vi "grSim_ReplacementTester.vi"(0 "Generate new random points":bool, 1 "IA State":T3, 2 "Atacando contra?":bool, 3 "Test Attacker":bool, 4 "id":i32, 5 "Field defense":i32[](array[numeric]), 6 "Test Mode On":bool, 7 "Number of Points":i32, 10 "Modulo Velocidade":dbl format="%#_13g", 11 "Test Passe":bool, 12 "reset":bool, 13 "Replace Robots":bool) -> (14 "grSim replacement":cluster{"robots":T1[], "ball":T2}, 15 "Replace active":bool, 18 "kick num":i32, 19 "Completed Generation":bool)   [LabVIEW 2017]
uses:
  Core/AI Input.ctl
  Core/AI Robot.ctl
  Intel/Functions Enum.ctl
  Intel/AttackerStates.ctl
  Path Planning/RRT/PathDests.ctl
  Path Planning/RRT/PathDest.ctl
  Core/AI Ball.ctl
  Core/Field Size.ctl
  Core/AI Judge.ctl
  Intel/Command Enum.ctl
  Util/Events/Events.ctl
  grSim RobotReplacement.ctl
  grSim_BallReplacement.ctl
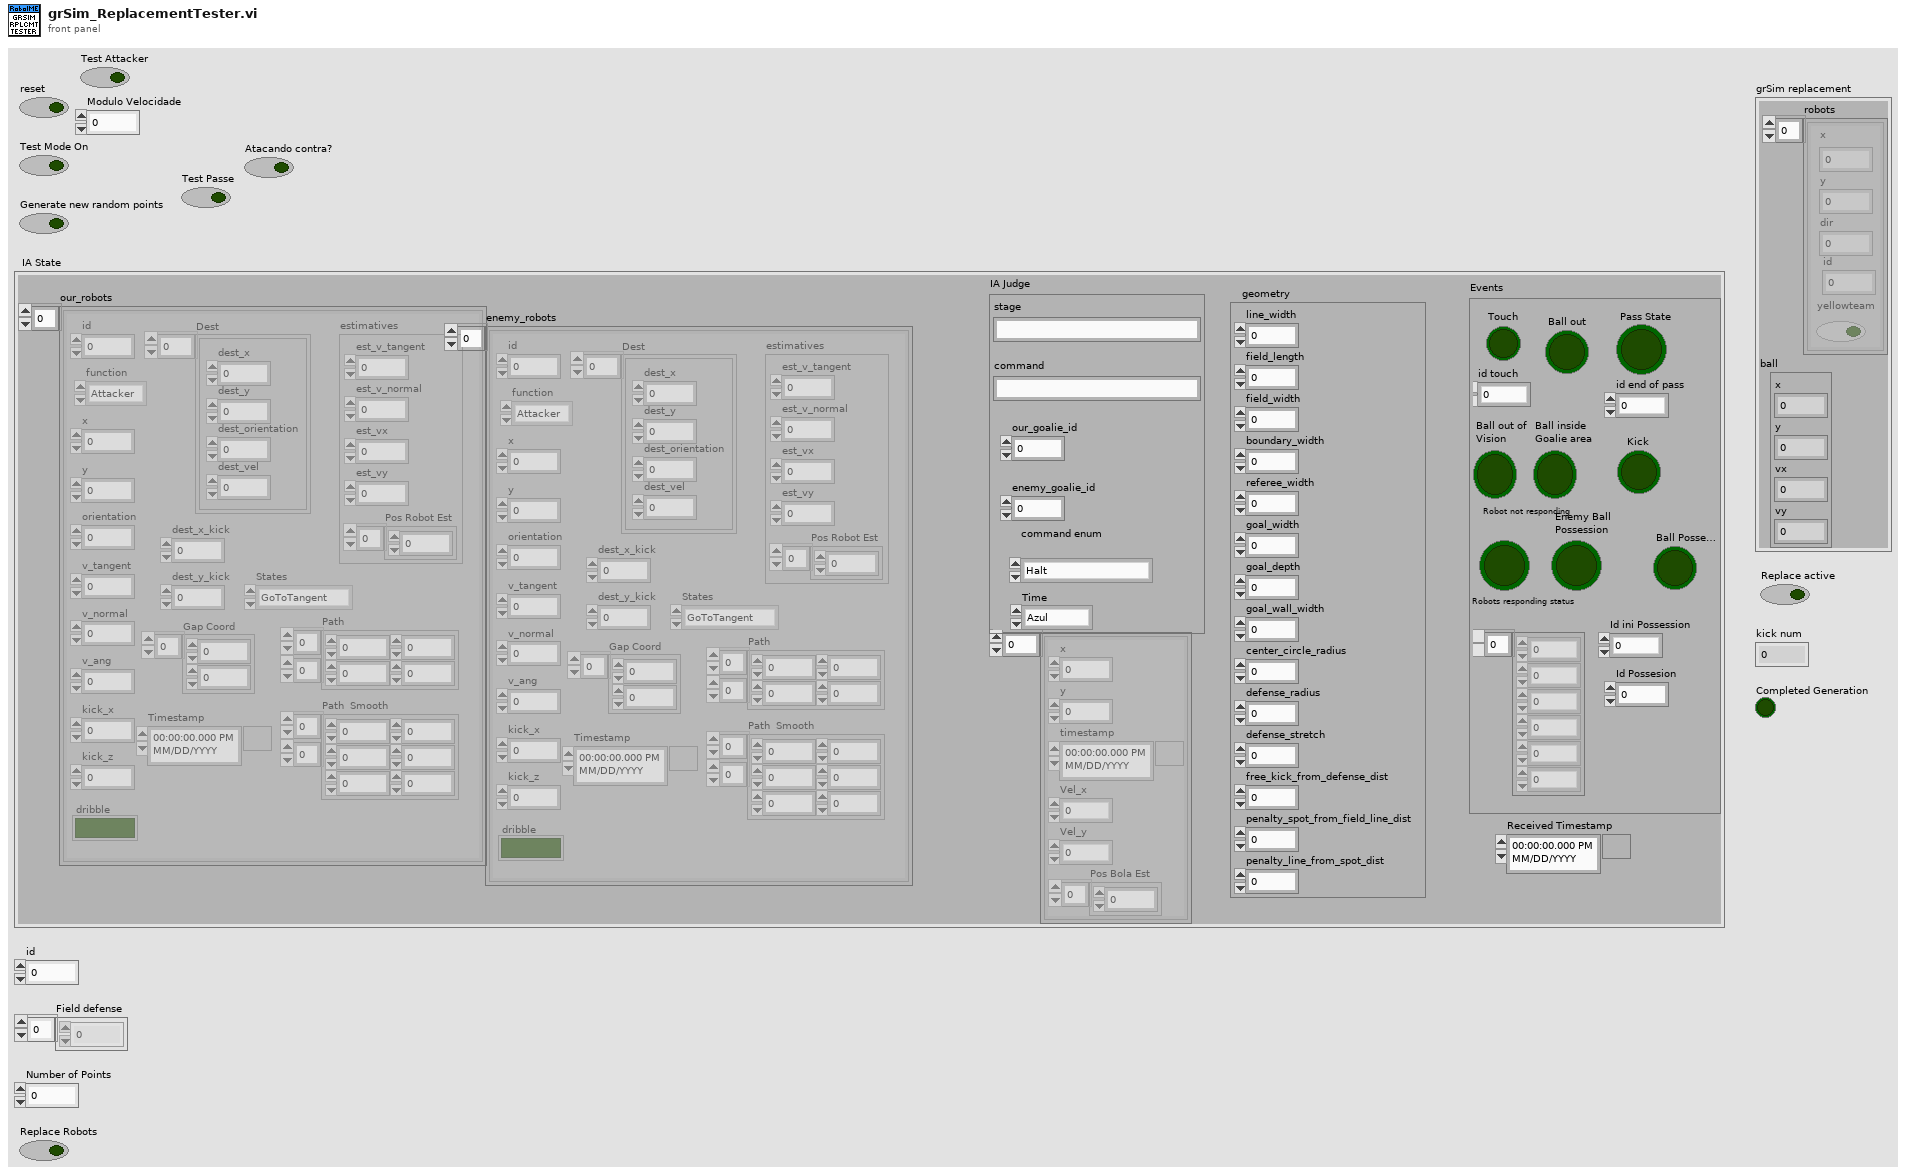
[diagram p1: front panel]
types:
  T1 = typedef "grSim RobotReplacement.ctl" = cluster{"x":dbl, "y":dbl, "dir":dbl, "yellowteam":bool, "id":u32}
  T2 = typedef "grSim_BallReplacement.ctl" = cluster{"x":dbl, "y":dbl, "vx":dbl, "vy":dbl}
  T3 = typedef "AI Input.ctl" = cluster{"our_robots":T4[], "enemy_robots":T4[], "balls":T9[], "geometry":T10, "IA Judge":T11, "Received Timestamp":timestamp, "Events":T13}
  T4 = typedef "AI Robot.ctl" = cluster{"id":u32, "function":T5, "x":dbl, "y":dbl, "orientation":dbl, "v_tangent":dbl, "v_normal":dbl, "v_ang":dbl, "kick_x":dbl, "kick_z":dbl, "dribble":bool, "Timestamp":timestamp, "estimatives":cluster{"est_v_tangent":dbl, "est_v_normal":dbl, "est_vx":dbl, "est_vy":dbl, "Pos Robot Est":dbl[]}, "dest_x_kick":dbl, "dest_y_kick":dbl, "Gap Coord":dbl[], "States":T6, "Path ":dbl[][], "Path  Smooth":dbl[][], "Dest":T7}
  T5 = typedef "Functions Enum.ctl" = enum16{"Attacker", "Goalie", "Defender", "Striker", "Goto 0", "Dummy", "Kicker", "ZigZag"}
  T6 = typedef "AttackerStates.ctl" = enum16{"Pass", "GoToTangent", "BallGetting", "GoToKick", ""}
  T7 = typedef "PathDests.ctl" = T8[]
  T8 = typedef "PathDest.ctl" = cluster{"dest_x":dbl, "dest_y":dbl, "dest_orientation":dbl, "dest_vel":dbl}
  T9 = typedef "AI Ball.ctl" = cluster{"x":dbl, "y":dbl, "timestamp":timestamp, "Vel_x":dbl, "Vel_y":dbl, "Pos Bola Est":dbl[]}
  T10 = typedef "Field Size.ctl" = cluster{"line_width":u32, "field_length":u32, "field_width":u32, "boundary_width":u32, "referee_width":u32, "goal_width":u32, "goal_depth":u32, "goal_wall_width":u32, "center_circle_radius":u32, "defense_radius":u32, "defense_stretch":u32, "free_kick_from_defense_dist":u32, "penalty_spot_from_field_line_dist":u32, "penalty_line_from_spot_dist":u32}
  T11 = typedef "AI Judge.ctl" = cluster{"stage":string, "command":string, "our_goalie_id":dbl, "enemy_goalie_id":dbl, "command enum":T12, "Time":enum16{"Azul", "Amarelo"}}
  T12 = typedef "Command Enum.ctl" = enum16{"Halt", "Stop", "Force Start", "PKA Normal Start", "Prepare Kickoff Ally", "PKE Normal Start", "Prepare Kickoff Enemy", "Prepare Penalty Ally", "PPA Normal Start", "Prepare Penalty Enemy", "PPE Normal Start", "Direct Free Enemy", "Direct Free Ally", "Indirect Free Enemy", "Indirect Free Ally", "Timeout Enemy", "Timeout Ally", "Goal Enemy", "Goal Ally", "Ball Placement Enemy", "Ball Placement Ally", "Normal Half Time", "Extra Time Break", "Extra Half Time", "None", "Post Game"}
  T13 = typedef "Events.ctl" = cluster{"Touch":bool, "Ball out":bool, "id touch":dbl, "Ball out of \nVision":bool, "Ball inside \nGoalie area":bool, "Robot not responding":bool, "Robots responding status":dbl[], "Enemy Ball \nPossession":bool, "Pass State":bool, "id end of pass":dbl, "Kick":bool, "Id ini Possession":dbl, "Ball Possesion":bool, "Id Possesion":dbl}
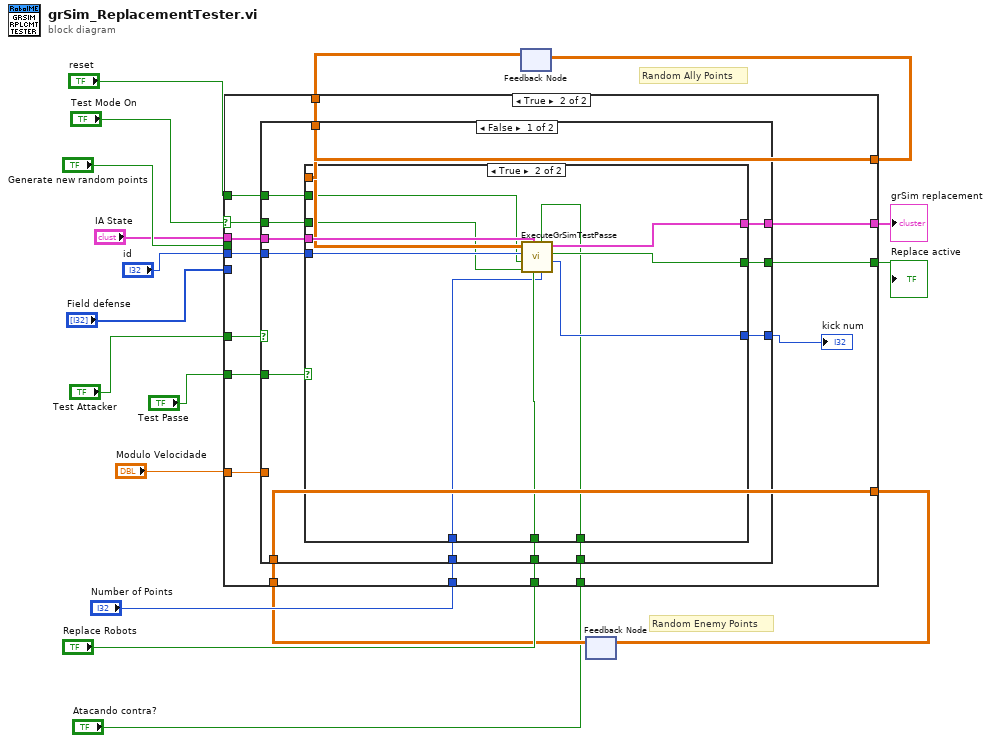
[diagram p0: block diagram]
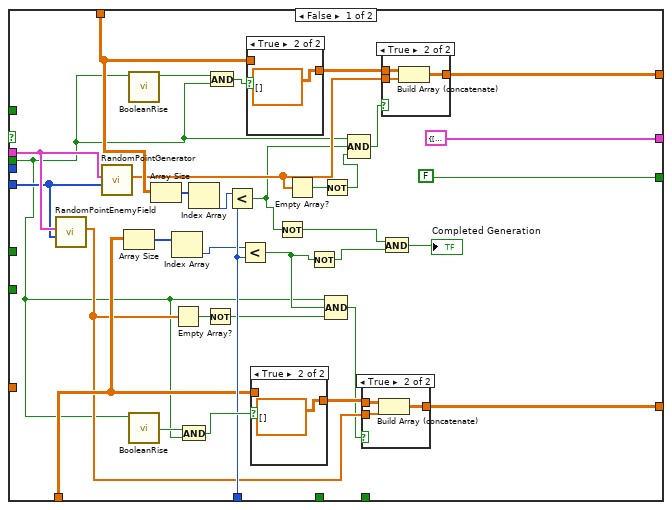
[diagram p2: hidden frame]
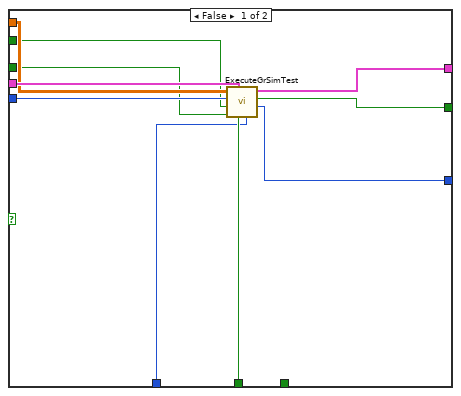
[diagram p7: hidden frame]
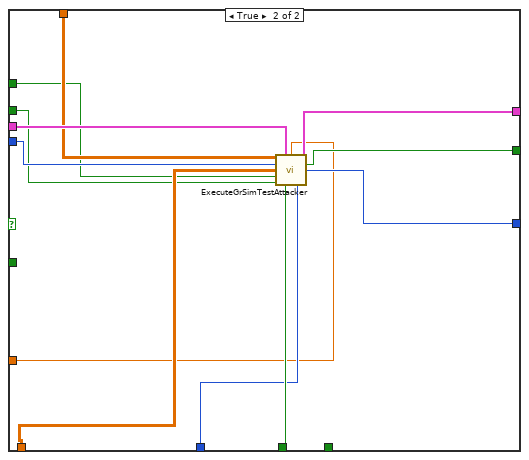
[diagram p8: hidden frame]
diagram:
  # "Random Enemy Points"
  # "Random Ally Points"
  n1 = feedback #1() -> (w14:dbl[][])  [unwired: 1 in]
  n2 = feedback #2() -> (w5:dbl[][])  [unwired: 1 in]
  n3 = case shown="True" "Test Mode On" {
    selector: "Test Mode On" -> [_ w73]
    tunnel: [cluster{"robots":T1[], "ball":T2} {"robots"=[], "ball"={"x"=0.0, "y"=0.0, "vx"=0.0, "vy"=0.0}} ("grSim replacement") w75] -> w7
    tunnel: [FALSE ("Replace active") w76] -> w8
    tunnel: "IA State" -> [w32 w78]
    tunnel: "Field defense" -> [w31 _]
    tunnel: "id" -> [_ w77]
    tunnel: "Generate new random points" -> [w19 _]
    tunnel: [w49 w74] -> w13
    tunnel: w14 -> [w46 w74]
    tunnel: "Number of Points" -> [w33 w70]
    tunnel: "reset" -> [_ w72]
    tunnel: "Replace Robots" -> [_ w71]
    tunnel: [w34 w67] -> w6
    tunnel: w5 -> [w30 w67]
    tunnel: "Test Attacker" -> [_ w69]
    tunnel: "Modulo Velocidade" -> [_ w68]
    tunnel: "Test Passe" -> [_ w65]
    tunnel: "Atacando contra?" -> [_ w64]
    frame False {
      n4 = call "RandomPointEnemyField.vi"("Field defense"=w31, "IA State Input"=w32) -> ("Point Enemy Field"=w29:dbl[])  [unwired: 9 in]
      n5 = call "RandomPointGenerator.vi"("Field defense"=w31, "IA State Input"=w32) -> ("Point Ally Field"=w42:dbl[])  [unwired: 9 in]
      n6 = Array Size(array=w30) -> (size(s)=w25:i32[])
      n7 = call "BooleanRise.vi"("Test Mode On"=w19) -> ("Boolean"=w38:bool)  [unwired: 10 in]
      n8 = call "BooleanRise.vi"("Test Mode On"=w19) -> ("Boolean"=w37:bool)  [unwired: 10 in]
      n9 = Array Size(array=w46) -> (size(s)=w44:i32[])
      n10 = Index Array(array=w25) -> (element=w24:i32)  [unwired: 1 in]
      n11 = Empty Array?(array=w29) -> (empty?=w28:bool)
      n12 = And(x=w37, y=w19) -> (x .and. y?=w36:bool)
      n13 = Index Array(array=w44) -> (element=w45:i32)  [unwired: 1 in]
      n14 = Not(x=w28) -> (.not. x?=w27:bool)
      n15 = And(x=w38, y=w19) -> (x .and. y?=w48:bool)
      n16 = Less?(x=w45, y=w33) -> (x < y?=w39:bool)
      n17 = Less?(x=w24, y=w33) -> (x < y?=w23:bool)
      n18 = case shown="True" w48 {
        tunnel: w46 -> [w62 _]
        tunnel: [w62 dbl[][] []] -> w47
        frame False {
        }
        frame True {
        }
      }
      n19 = case shown="True" w36 {
        tunnel: [w56 dbl[][] []] -> w35
        tunnel: w30 -> [w56 _]
        frame False {
        }
        frame True {
        }
      }
      n20 = Not(x=w39) -> (.not. x?=w22:bool)
      n21 = Empty Array?(array=w42) -> (empty?=w40:bool)
      n22 = Not(x=w23) -> (.not. x?=w21:bool)
      n23 = Not(x=w40) -> (.not. x?=w41:bool)
      n24 = Compound Arithmetic op=AND(w19, w23, w27) -> (w26:bool)
      n25 = Compound Arithmetic op=AND(w19, w39, w41) -> (w43:bool)
      n26 = case shown="True" w26 {
        tunnel: [w52 w55] -> w34
        tunnel: w35 -> [w52 w54]
        tunnel: w29 -> [_ w53]
        frame False {
        }
        frame True {
          n27 = Build Array (concatenate)(w54, w53) -> (w55:dbl[][])
        }
      }
      n28 = case shown="True" w43 {
        tunnel: w42 -> [_ w61]
        tunnel: [w58 w60] -> w49
        tunnel: w47 -> [w58 w59]
        frame False {
        }
        frame True {
          n29 = Build Array (concatenate)(w59, w61) -> (w60:dbl[][])
        }
      }
      n30 = And(x=w22, y=w21) -> (x .and. y?=→"Completed Generation":bool)
    }
    frame True {
      n31 = case shown="False" w69 {
        tunnel: w78 -> [w90 w123]
        tunnel: w77 -> [w89 w120]
        tunnel: [w88 w115] -> w76
        tunnel: [w87 w114] -> w75
        tunnel: w74 -> [w86 w122]
        tunnel: w73 -> [w85 w118]
        tunnel: w72 -> [w84 w119]
        tunnel: w71 -> [w83 w117]
        tunnel: w70 -> [w82 w116]
        tunnel: w68 -> [_ w112]
        tunnel: w67 -> [_ w121]
        tunnel: [w81 w113] -> w66
        tunnel: w65 -> [w80 _]
        tunnel: w64 -> [w79 _]
        frame False {
          n32 = case shown="True" w80 {
            tunnel: w90 -> [w100 w111]
            tunnel: w89 -> [w99 w110]
            tunnel: [w98 w109] -> w88
            tunnel: [w97 w108] -> w87
            tunnel: w86 -> [w96 w107]
            tunnel: w85 -> [w95 w106]
            tunnel: w84 -> [w94 w105]
            tunnel: w83 -> [w93 w104]
            tunnel: w82 -> [w92 w103]
            tunnel: [w91 w102] -> w81
            tunnel: w79 -> [_ w101]
            frame False {
              n33 = call "ExecuteGrSimTest.vi"("Number of Points"=w92, "Replace Robots"=w93, "IA State Input"=w100, "Test Mode On"=w95, "reset"=w94, "id"=w99, "RandomAllyPoints"=w96) -> ("kick num"=w91:i32, "Replace active"=w98:bool, "grSim replacement"=w97:cluster{"robots":T1[], "ball":T2})  [unwired: 2 in]
            }
            frame True {
              n34 = call "ExecuteGrSimTestPasse.vi"("Number of Points"=w103, "Atacando contra?"=w101, "Replace Robots"=w104, "IA State Input"=w111, "Test Mode On"=w106, "reset"=w105, "id"=w110, "RandomAllyPoints"=w107) -> ("kick num"=w102:i32, "Replace active"=w109:bool, "grSim replacement"=w108:cluster{"robots":T1[], "ball":T2})  [unwired: 1 in]
            }
          }
        }
        frame True {
          n35 = call "ExecuteGrSimTestAttacker.vi"("RandomAllyPoints"=w122, "IA State Input"=w123, "Modulo Velocidade"=w112, "id"=w120, "RandomEnemyPoints"=w121, "reset"=w119, "Test Mode On"=w118, "Replace Robots"=w117, "Number of Points"=w116) -> ("grSim replacement"=w114:cluster{"robots":T1[], "ball":T2}, "Replace active"=w115:bool, "kick num"=w113:i32)  [unwired: 4 in]
        }
      }
      "kick num" <- w66
    }
  }
  "Replace active" <- w8
  "grSim replacement" <- w7
  n36 = feedback-in #1(w13) -> ()
  n37 = feedback-in #2(w6) -> ()
